vi "SVT Weighting Filter.vi"   [LabVIEW 2017, in "SoundVib_ABCWeighting.lvlib"]
doc: "Applies the selected weighting to <B>scaled signal [EU]</B>. This VI complies with ANSI S1.4-1983, ANSI S1.42-2001, IEC 61672-1:2002, and JIS C 1509-1:2005 standards. Use Each instance of this VI maintains its own state; use the N Channel instance of this VI to process an array of channels. This VI operates on time-continuous data; it resets on a discontinuity. Wire data to the <B>scaled signal [EU]</B> input to determine the polymorphic instance to use or manually select the instance."
uses:
  <vilib>/addons/Sound and Vibration/svt_Weighting/SoundVib_ABCWeighting.lvlib
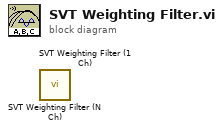
[diagram p0: block diagram]
diagram:
  n1 = call <vilib>:"SVT Weighting Filter (N Ch).vi"() -> ()  [unwired: 9 in, 2 out]
  n2 = call <vilib>:"SVT Weighting Filter (1 Ch).vi"() -> ()  [unwired: 9 in, 2 out]
